vi "token--image.vi"() -> ()   [LabVIEW 2021]
panel:
  in  "template--token":bool
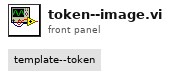
[diagram p1: front panel]
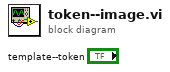
[diagram p0: block diagram]
diagram:
